vi "Node - PXImc Open.vi"(8 "error in (no error)":errorcluster, 11 "Node Data In in":T1) -> (0 "error out":errorcluster, 3 "Node Data In out":T1)   [LabVIEW 2016, in "PXImc Router.lvlib"]
uses:
  PXImc Router.lvlib
  Controls/Node Data.ctl
  Controls/Node/Node - PXImc Parameters.ctl
  Controls/Node/Node - Writer Data.ctl
  Controls/Node/Node Ch Properties.ctl
  Controls/Data Type.ctl
  Controls/Node/Node - Readers Data.ctl
  Controls/Node/Node - Reader Data.ctl
  <vilib>/pximc/Initialize Writer Session (U8).vi
  <vilib>/pximc/Initialize Reader Session (U8).vi
  <vilib>/pximc/nipximc.lvlib
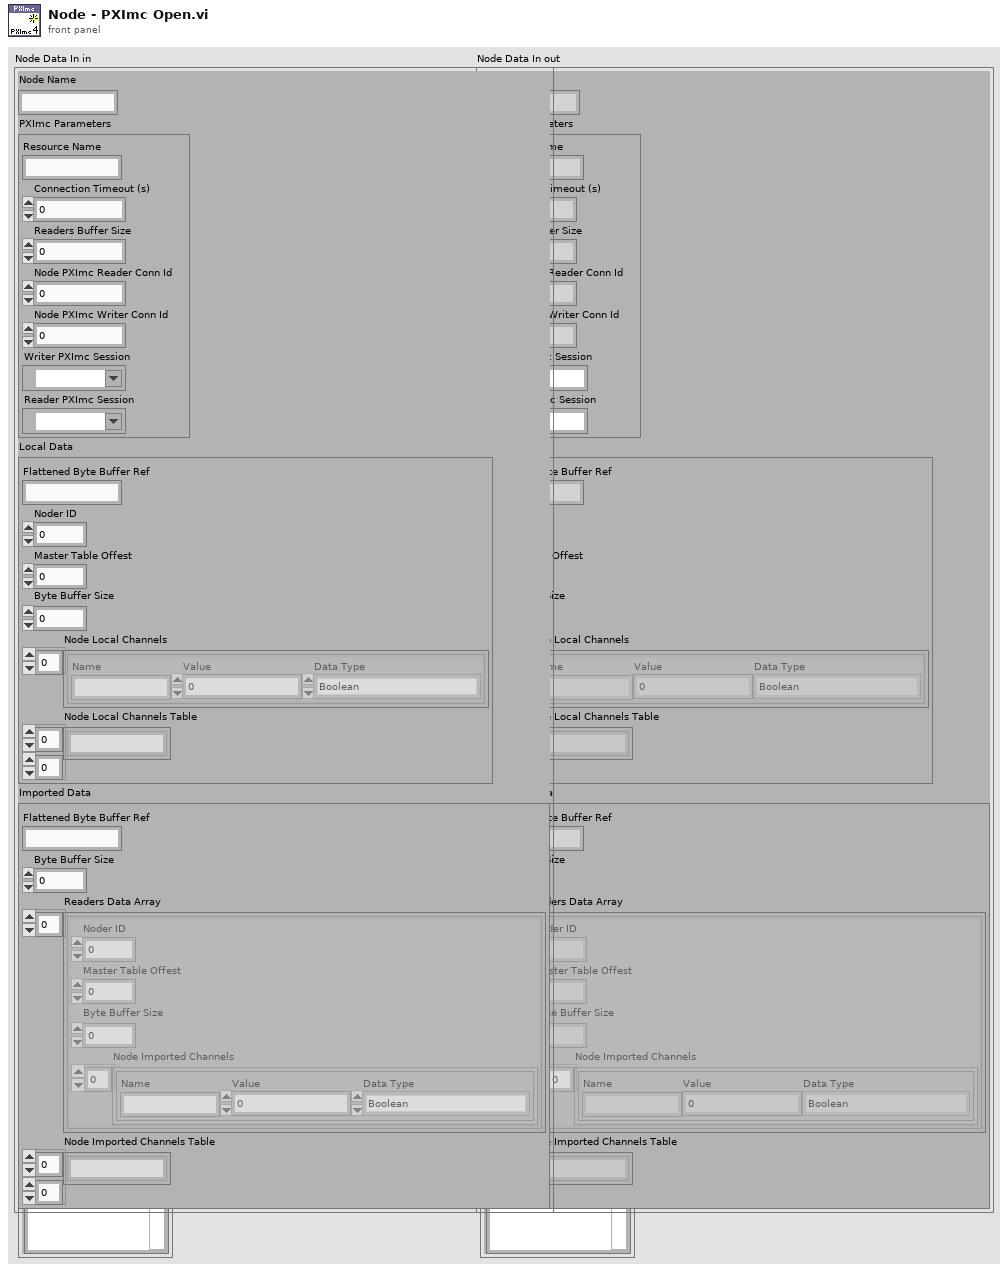
[diagram p1: front panel]
types:
  T1 = typedef "PXImc Router.lvlib/Node Data.ctl" = cluster{"Node Name":string, "PXImc Parameters":T2, "Local Data":T3, "Imported Data":T6}
  T2 = typedef "PXImc Router.lvlib/Node - PXImc Parameters.ctl" = cluster{"Resource Name":string, "Connection Timeout (s)":dbl, "Readers Buffer Size":u64, "Node PXImc Reader Conn Id":u16, "Node PXImc Writer Conn Id":u16, "Writer PXImc Session":refnum<k21>, "Reader PXImc Session":refnum<k21>}
  T3 = typedef "PXImc Router.lvlib/Node - Writer Data.ctl" = cluster{"Flattened Byte Buffer Ref":string, "Noder ID":u32, "Master Table Offest":u32, "Byte Buffer Size":u32, "Node Local Channels":T4[], "Node Local Channels Table":string[][]}
  T4 = typedef "PXImc Router.lvlib/Node Ch Properties.ctl" = cluster{"Name":string, "Value":dbl, "Data Type":T5}
  T5 = typedef "PXImc Router.lvlib/Data Type.ctl" = enum16{"Boolean", "SGL", "DBL", "I8", "I16", "I32", "I64", "U8", "U16", "U32", "U64"}
  T6 = typedef "PXImc Router.lvlib/Node - Readers Data.ctl" = cluster{"Flattened Byte Buffer Ref":string, "Byte Buffer Size":u64, "Readers Data Array":T7[], "Node Imported Channels Table":string[][]}
  T7 = typedef "PXImc Router.lvlib/Node - Reader Data.ctl" = cluster{"Noder ID":u32, "Master Table Offest":u32, "Byte Buffer Size":u64, "Node Imported Channels":T4[]}
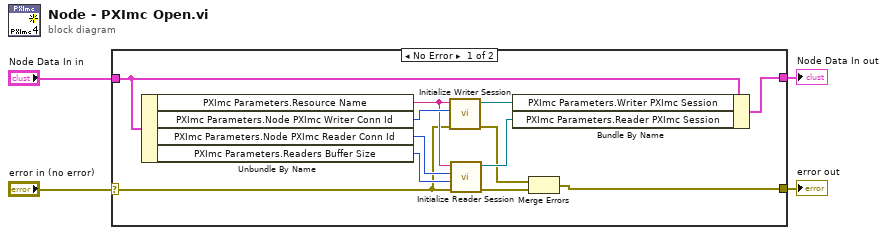
[diagram p0: block diagram]
diagram:
  n1 = case shown="No Error" "error in (no error)" {
    selector: "error in (no error)" -> [w6 w17]
    tunnel: "Node Data In in" -> [w5 w18]
    tunnel: [w9 w18] -> w2
    tunnel: [w16 w17] -> w4
    frame No Error {
      n2 = Unbundle By Name(w5) -> ("PXImc Parameters.Resource Name"=w12:string, "PXImc Parameters.Node PXImc Writer Conn Id"=w15:u16, "PXImc Parameters.Node PXImc Reader Conn Id"=w13:u16, "PXImc Parameters.Readers Buffer Size"=w11:u64)
      n3 = call-poly <vilib>:"Initialize Writer Session.vi"("error in (no error)"=w6, "connection id (1)"=w15, "interface"=w12) -> ("error out"=w8:errorcluster, "session out"=w14:refnum<k21>)  [unwired: 7 in]
      n4 = call-poly <vilib>:"Initialize Reader Session.vi"("error in (no error)"=w6, "buffer size"=w11, "writer's connection id (1)"=w13, "interface"=w12) -> ("error out"=w7:errorcluster, "session out"=w10:refnum<k21>)  [unwired: 6 in]
      n5 = Bundle By Name(cluster=w5, "PXImc Parameters.Writer PXImc Session"=w14, "PXImc Parameters.Reader PXImc Session"=w10) -> (w9:T1)
      n6 = Merge Errors(w8, w7) -> (w16:errorcluster)
    }
    frame Error {
    }
  }
  "error out" <- w4
  "Node Data In out" <- w2
